vi "get waveform.vi"(8 "error in (no error)":errorcluster caption="에러 입력(에러 없음)", 11 "WAV File 입력":refnum<class "WAV File.lvclass">) -> (0 "error out":errorcluster caption="에러 출력", 2 "waveform":waveform(dbl), 3 "WAV File 출력":refnum<class "WAV File.lvclass">)   [LabVIEW 2020, in "WAV File.lvclass"]
uses:
  WAV File.lvclass
  Waveform Obj/Waveform Obj.lvclass/Waveform Obj.ctl
  Waveform Obj/Accessors/Read sampling rate.vi
  <vilib>/measure/maresamp.llb/Resample Waveform (single shot).vi
  <vilib>/measure/NI_MAPro.lvlib
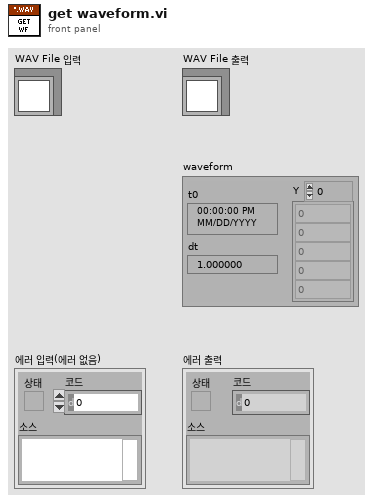
[diagram p1: front panel]
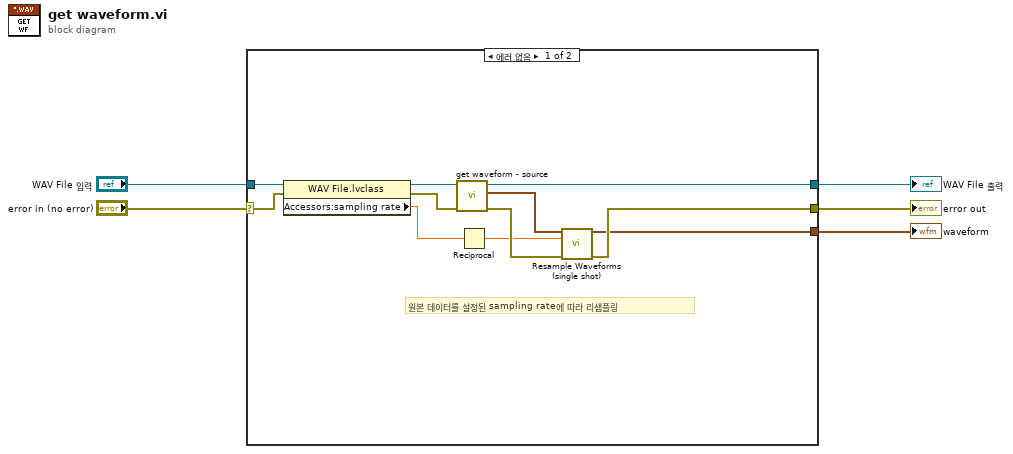
[diagram p0: block diagram]
diagram:
  n1 = case shown="에러 없음" "error in (no error)" {
    selector: "error in (no error)" -> [w16 w18]
    tunnel: [w7 w18] -> w4
    tunnel: "WAV File 입력" -> [w11 w17]
    tunnel: [w15 w17] -> w2
    tunnel: [w6 _] -> w1
    frame No Error {
      # "원본 데이터를 설정된 sampling rate에 따라 리샘플링"
      n2 = property class="WAV File.lvclass"(reference=w11, error in=w16) -> (reference out=w10:refnum<class "WAV File.lvclass">, error out=w12:errorcluster, "Accessors:sampling rate"=w9:dbl)
      n3 = call-dynamic "get waveform - source.vi"("error in (no error)"=w12, "WAV File 입력"=w10) -> ("error out"=w13:errorcluster, "waveform"=w14:waveform(dbl), "WAV File 출력"=w15:refnum<class "WAV File.lvclass">)  [unwired: 7 in]
      n4 = Reciprocal(x=w9) -> (1/x=w8:dbl)
      n5 = call-poly <vilib>:"Resample Waveforms (single shot).vi"("waveform in"=w14, "dt"=w8, "error in (no error)"=w13) -> ("resampled waveform out"=w6:waveform(dbl), "error out"=w7:errorcluster)  [unwired: 9 in, 2 out]
    }
    frame Error {
    }
  }
  "error out" <- w4
  "WAV File 출력" <- w2
  "waveform" <- w1
